vi "configure resonance PXI.vi"(6 "x resonant zoom voltage":dbl, 8 "error in":errorcluster, 9 "y-voltage":dbl=2.0, 10 "Start Delay (Ticks)":i16, 11 "lines (2pi) per frame":i32=100) -> (0 "error out":errorcluster, 1 "pixels per frame":dbl, 2 "FPGA VI Reference Out":refnum<k20>, 3 "AO task out":refnum<k21>, 4 "Actual Depth":u32)   [LabVIEW 2012]
uses:
  <vilib>/rvi/interface/nirviOpenFPGA/nirviOpenFPGA.xnode
  <vilib>/rvi/interface/nirviMethod/nirviMethod.xnode
  <vilib>/rvi/interface/nirviReadWriteControl/nirviReadWriteControl.xnode
  <vilib>/rvi/errors/niLvFpgaMergeErrorWithErrorCode.vi
  <vilib>/DAQmx/create/channels.llb/DAQmx Create Channel (AO-Voltage-Basic).vi
  <vilib>/DAQmx/configure/timing.llb/DAQmx Timing (Sample Clock).vi
  <vilib>/DAQmx/configure/trigger.llb/DAQmx Start Trigger (Digital Edge).vi
  <vilib>/DAQmx/write.llb/DAQmx Write (Analog 2D DBL NChan NSamp).vi
  GFG/GFG library.lvlib
  GFG/GFGbooleanGet.vi
  GFG/GFGnumericGet.vi
  GFG/GFGfpRefGet.vi
  FPGA/current bitfiles/4chresonancescan_PXIe-7962R_newLindsaymod4ch_VaUfink3TSc.lvbitx
  <vilib>/FPGAPlugInAG/PXIe-7962R/niLvFpga_ConfigureFifo_PXIe-7962R.vi
  <vilib>/FPGAPlugInAG/PXIe-7962R/niLvFpga_ReadFifo_PXIe-7962R.vi
  <vilib>/FPGAPlugInAG/PXIe-7962R/niLvFpga_Open_PXIe-7962R.vi
  <vilib>/FPGAPlugInAG/PXIe-7962R/niLvFpga_Abort_PXIe-7962R.vi
  NiFpgaLv.dll
  <vilib>/Utility/error.llb/Error Cluster From Error Code.vi
  <vilib>/rvi/errors/niLvFpgaAdjustHostInterfaceError.vi
  <vilib>/FPGAPlugInAG/PXIe-7962R/niLvFpga_Run_PXIe-7962R.vi
  <vilib>/userDefined/High Color/nirio_resource_hc.ctl
panel:
  out "Waveform Graph":dbl[][](graph)
  in  "Requested Depth":u32=10000000
  out "Actual Depth 3":u32
  in  "RIO Device":T1="RIO0"
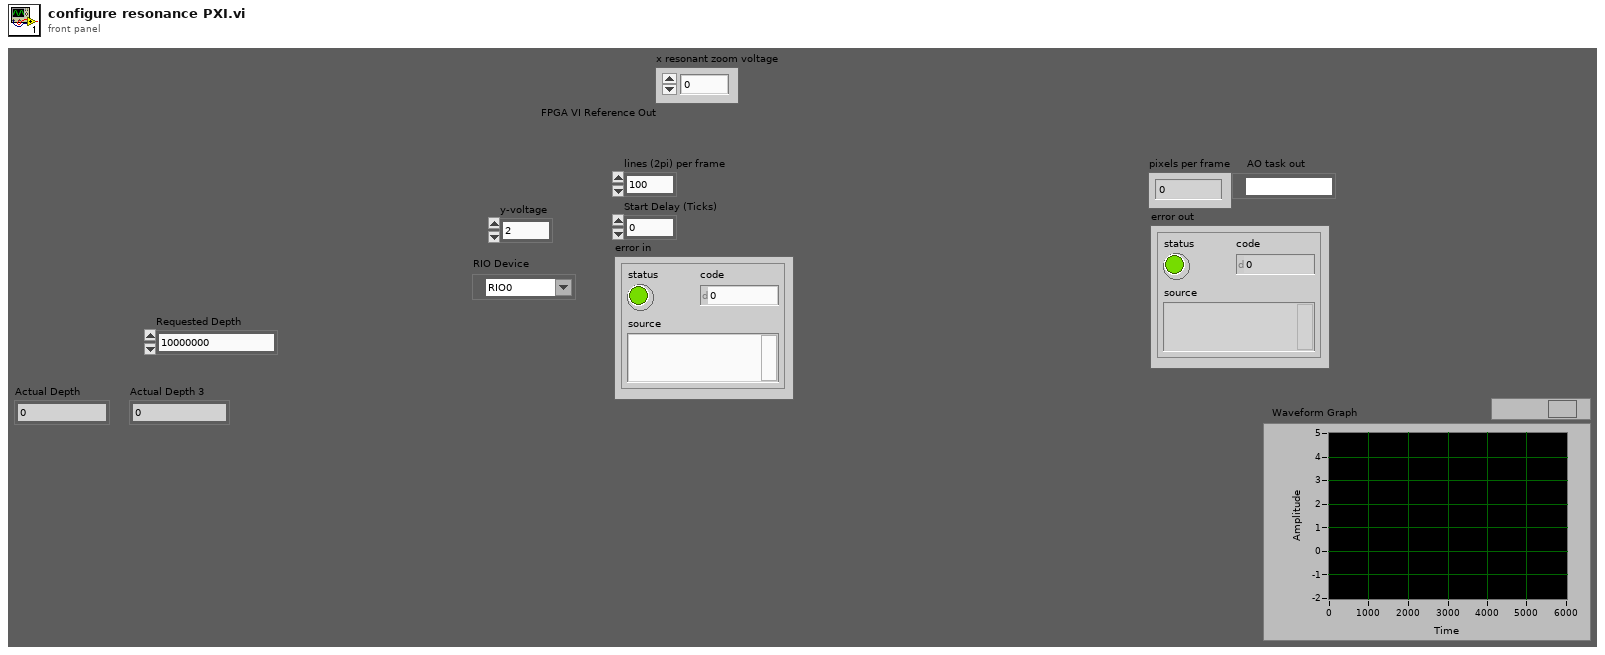
[diagram p1: front panel]
types:
  T1 = typedef "nirio_resource_hc.ctl" = tag
  T2 = enum8{"Enabled", "Disabled", "Disabled and Grayed Out"}
  T3 = cluster{"WaveformChartRef":refnum<vi>, "DigitalRef":refnum<vi>, "ArrayRef":refnum<vi>, "TabControlRef":refnum<vi>, "EnumRef":refnum<vi>, "RingRef":refnum<vi>, "BooleanRef":refnum<vi>, "KnobRef":refnum<vi>, "SlideRef":refnum<vi>, "PathRef":refnum<vi>, "StringRef":refnum<vi>, "ComboBox":refnum<vi>, "WaveformGraphRef":refnum<vi>}
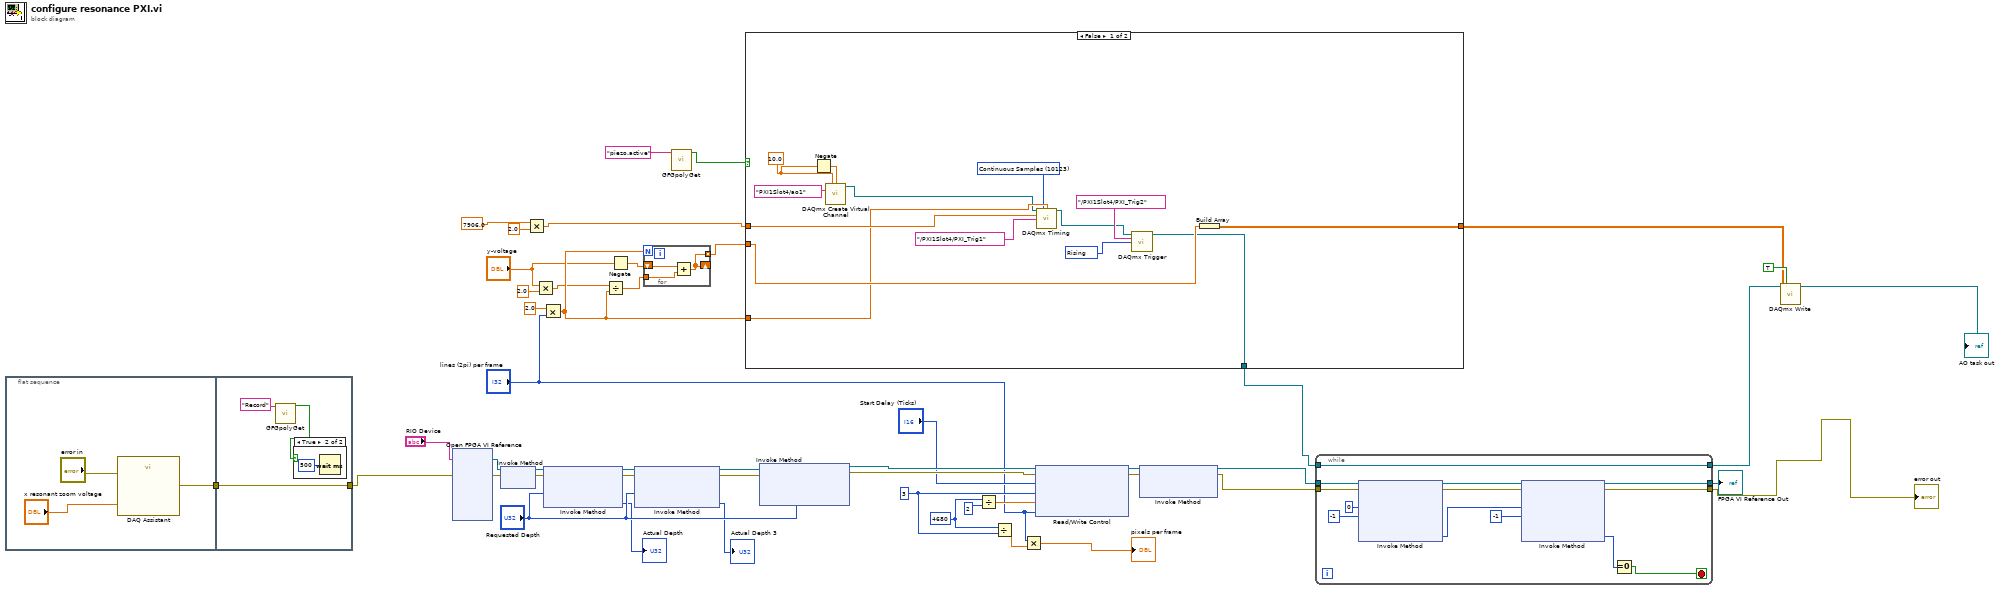
[diagram p0: block diagram]
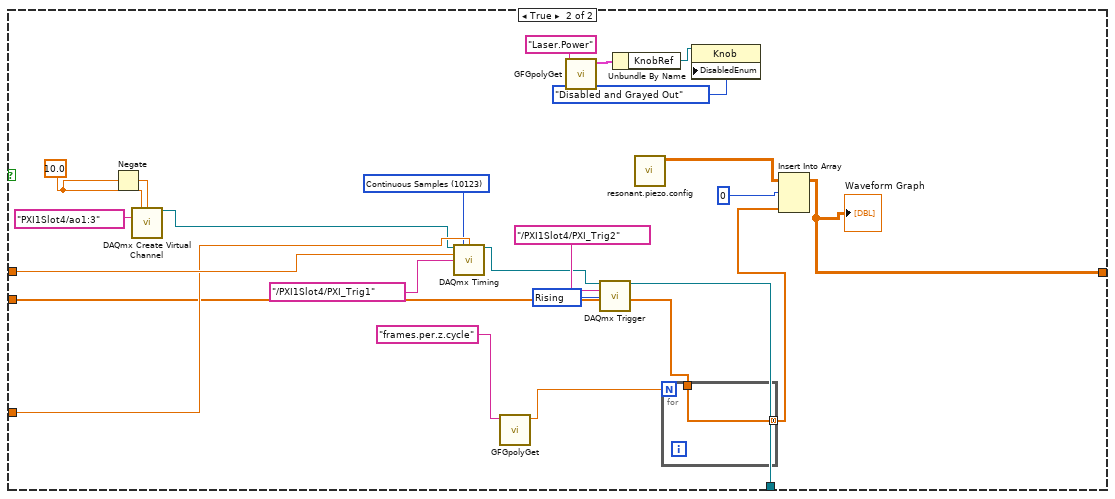
[diagram p3: hidden frame]
diagram:
  w41 = 3 ("dwell time in ticks")
  w37 = i16 4680 ("samples per period")
  n1 = flat-sequence {
    tunnel: [w49] -> w2
    tunnel: [w54] -> w13
    tunnel: w2 -> [w54]
    frame #0 {
      n2 = call "DAQ Assistant"("data"="x resonant zoom voltage", "error in"="error in") -> ("error out"=w49:errorcluster)  [unwired: 16 in, 1 out]
    }
    frame #1 {
      n3 = call-poly "GFGpolyGet.vi"("Variable Name in"="Record") -> ("Boolean"=w52:bool)  [unwired: 10 in]
      n4 = case shown="True" w52 {
        frame False {
        }
        frame True {
          n5 = Wait (ms)(milliseconds to wait=u32 500) -> ()  [unwired: 1 out]
        }
      }
    }
  }
  n6 = xnode "Open FPGA VI Reference"("error in"=w13, "resource name"="RIO Device") -> ("FPGA VI Reference Out"=w46:refnum<k20>, "error out"=w47:errorcluster)
  n7 = xnode "Invoke Method"("FPGA VI Reference In"=w46, "error in"=w47) -> ("FPGA VI Reference Out"=w45:refnum<k20>, "error out"=w43:errorcluster)
  n8 = Multiply(x=7906.0 ("rate"), y=2.0) -> (x*y=w27:dbl)
  n9 = Multiply(x="y-voltage", y=2.0) -> (x*y=w21:dbl)
  n10 = Multiply(x=2.0, y="lines (2pi) per frame") -> (x*y=w26:dbl)
  n11 = xnode "Invoke Method"("FPGA VI Reference In"=w45, "error in"=w43, "Requested Depth"="Requested Depth") -> ("FPGA VI Reference Out"=w7:refnum<k20>, "error out"=w6:errorcluster, "Actual Depth"=→"Actual Depth":u32)
  n12 = Divide(x=w21, y=w26) -> (x/y=w17:dbl)
  n13 = Negate(x="y-voltage") -> (-x=w18:dbl)
  n14 = xnode "Invoke Method"("FPGA VI Reference In"=w7, "error in"=w6, "Requested Depth"="Requested Depth") -> ("FPGA VI Reference Out"=w5:refnum<k20>, "error out"=w4:errorcluster, "Actual Depth"=→"Actual Depth 3":u32)
  n15 = for {
    N: w26 -> [_]
    tunnel: w17 -> [w57]
    shift-right: [w56] -> _
    shift-left: w18 -> [w58]
    tunnel: [w56] -> w29 mode=indexing
    n16 = Add(x=w58, y=w57) -> (x+y=w56:dbl)
  }
  n17 = call-poly "GFGpolyGet.vi"("Variable Name in"="piezo.active") -> ("Boolean"=w10:bool)  [unwired: 10 in]
  n18 = case shown="False" w10 {
    tunnel: w29 -> [w72 w79]
    tunnel: w27 -> [w70 w94]
    tunnel: w26 -> [w67 w91]
    tunnel: [w61 w85] -> w16
    tunnel: [w59 w81] -> w12
    frame False {
      w71 = 10280 items=["Rising"=10280, "Falling"=10171] ("edge")
      w64 = 10123 items=["Finite Samples"=10178, "Continuous Samples"=10123, "Hardware Timed Single Point"=12522] ("sample mode")
      w65 = 10.0 ("maximum value")
      n19 = Negate(x=w65) -> (-x=w66:dbl)
      n20 = call-poly <vilib>:"DAQmx Create Virtual Channel.vi"("maximum value"=w65, "minimum value"=w66, "physical channels"=tag "PXI1Slot4/ao1") -> ("task out"=w62:refnum<k21>)  [unwired: 11 in, 1 out]
      n21 = call-poly <vilib>:"DAQmx Timing.vi"("task/channels in"=w62, "sample mode"=w64, "samples per channel"=w67, "rate"=w70, "source"=tag "/PXI1Slot4/PXI_Trig1") -> ("task out"=w60:refnum<k21>)  [unwired: 9 in, 1 out]
      n22 = call-poly <vilib>:"DAQmx Trigger.vi"("task/channels in"=w60, "source"=tag "/PXI1Slot4/PXI_Trig2", "edge"=w71) -> ("task out"=w61:refnum<k21>)  [unwired: 11 in, 1 out]
      n23 = Build Array(w72) -> (w59:dbl[][])
    }
    frame True {
      w95 = 10280 items=["Rising"=10280, "Falling"=10171] ("edge")
      w88 = 10123 items=["Finite Samples"=10178, "Continuous Samples"=10123, "Hardware Timed Single Point"=12522] ("sample mode")
      w89 = 10.0 ("maximum value")
      n24 = Negate(x=w89) -> (-x=w90:dbl)
      n25 = call-poly <vilib>:"DAQmx Create Virtual Channel.vi"("maximum value"=w89, "minimum value"=w90, "physical channels"=tag "PXI1Slot4/ao1:3") -> ("task out"=w86:refnum<k21>)  [unwired: 11 in, 1 out]
      n26 = call-poly <vilib>:"DAQmx Timing.vi"("task/channels in"=w86, "sample mode"=w88, "samples per channel"=w91, "rate"=w94, "source"=tag "/PXI1Slot4/PXI_Trig1") -> ("task out"=w84:refnum<k21>)  [unwired: 9 in, 1 out]
      n27 = call-poly "GFGpolyGet.vi"("Variable Name in"="frames.per.z.cycle" ("Tag in")) -> ("Numeric"=w78:dbl)  [unwired: 9 in, 1 out]
      n28 = call-poly "GFGpolyGet.vi"("Variable Name in"="Laser.Power") -> ("output cluster"=w76:T3)  [unwired: 9 in, 1 out]
      n29 = call-poly <vilib>:"DAQmx Trigger.vi"("task/channels in"=w84, "source"=tag "/PXI1Slot4/PXI_Trig2", "edge"=w95) -> ("task out"=w85:refnum<k21>)  [unwired: 11 in, 1 out]
      n30 = Unbundle By Name(w76) -> ("KnobRef"=w73:refnum<vi>)
      n31 = call "resonant.piezo.config.vi"() -> ("appended array"=w83:dbl[][])  [unwired: 11 in]
      n32 = for {
        N: w78 -> [_]
        tunnel: w79 -> [w96]
        tunnel: [w96] -> w77 mode=concatenating
      }
      n33 = property class="Knob"(reference=w73, "DisabledEnum"=T2."Disabled and Grayed Out" ("Disabled")) -> ()  [unwired: 1 in, 2 out]
      n34 = Insert Into Array(array=w83, index (row)=0 ("disabled index (col)"), new element=w77) -> (w81:dbl[][])  [unwired: 1 in]
      "Waveform Graph" <- w81
    }
  }
  n35 = xnode "Invoke Method"("FPGA VI Reference In"=w5, "error in"=w4, "Requested Depth"="Requested Depth") -> ("FPGA VI Reference Out"=w40:refnum<k20>, "error out"=w39:errorcluster)  [unwired: 1 out]
  n36 = Divide(x=w37, y=i16 2) -> (x/y=w35:dbl)
  n37 = Divide(x=w37, y=w41) -> (x/y=w33:dbl)
  n38 = Multiply(x="lines (2pi) per frame", y=w33) -> (x*y=→"pixels per frame":dbl)
  n39 = xnode "Read/Write Control"("FPGA VI Reference In"=w40, "error in"=w39, "Start Delay (Ticks)"="Start Delay (Ticks)", "dwell time in ticks"=w41, "samples per half period"=w35, "lines at once"="lines (2pi) per frame") -> ("FPGA VI Reference Out"=w44:refnum<k20>, "error out"=w42:errorcluster)
  n40 = xnode "Invoke Method"("FPGA VI Reference In"=w44, "error in"=w42) -> ("FPGA VI Reference Out"=w31:refnum<k20>, "error out"=w30:errorcluster)  [unwired: 1 in]
  n41 = while {
    tunnel: w31 -> [w109]
    tunnel: w30 -> [w101]
    tunnel: [w99] -> w1
    tunnel: [w98] -> w3
    tunnel: w16 -> [w97]
    tunnel: [w97] -> w14
    stop <- w102 stop-if-true
    n42 = xnode "Invoke Method"("FPGA VI Reference In"=w109, "error in"=w101, "Number of Elements"=u32 0, "Timeout (ms)"=-1) -> ("FPGA VI Reference Out"=w105:refnum<k20>, "error out"=w100:errorcluster, "Elements Remaining"=w104:u32)  [unwired: 1 out]
    n43 = xnode "Invoke Method"("FPGA VI Reference In"=w105, "error in"=w100, "Number of Elements"=w104, "Timeout (ms)"=-1) -> ("FPGA VI Reference Out"=w99:refnum<k20>, "error out"=w98:errorcluster, "Elements Remaining"=w103:u32)  [unwired: 1 out]
    n44 = Equal To 0?(x=w103) -> (x = 0?=w102:bool)
  }
  "error out" <- w3
  "FPGA VI Reference Out" <- w1
  n45 = call-poly <vilib>:"DAQmx Write.vi"("task/channels in"=w14, "auto start"=TRUE, "data"=w12) -> ("task out"=→"AO task out":refnum<k21>)  [unwired: 10 in, 2 out]
